vi "FaceEncoding.vi"(7 "numJitters":i32, 8 "error in (no error)":errorcluster, 9 "knownFaceLocation":refnum<k24>, 10 "image":refnum<k24>, 11 "FaceRecognition in":refnum<class "FaceRecognition.lvclass">) -> (0 "error out":errorcluster, 2 "FirstFaceEncoding":refnum<k24>, 3 "FaceRecognition out":refnum<class "FaceRecognition.lvclass">)   [LabVIEW 2020, in "FaceRecognitionDotNet.lvlib" / "FaceRecognition.lvclass"]
uses:
  FaceRecognition.lvclass
  dll/FaceRecognitionDotNet.dll
  FaceRecognition.lvclass/FaceRecognition.ctl
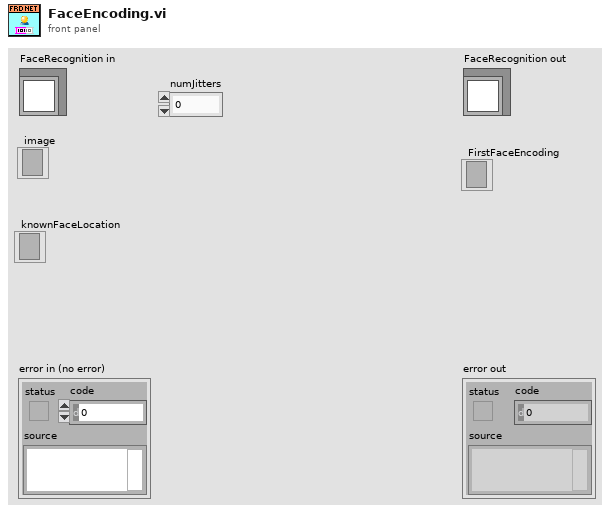
[diagram p1: front panel]
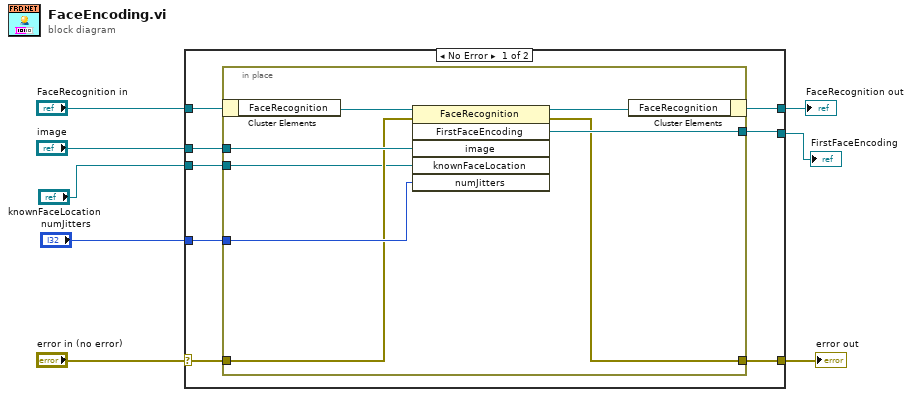
[diagram p0: block diagram]
diagram:
  n1 = case shown="No Error" "error in (no error)" {
    selector: "error in (no error)" -> [w14 w26]
    tunnel: [w13 w26] -> w7
    tunnel: [w15 w25] -> w5
    tunnel: "FaceRecognition in" -> [w16 w25]
    tunnel: [w12 _] -> w2
    tunnel: "image" -> [w11 _]
    tunnel: "numJitters" -> [w10 _]
    tunnel: "knownFaceLocation" -> [w9 _]
    frame No Error {
      n2 = in-place {
        in-place-border: w14 -> [w19]
        in-place-border: [w18] -> w13
        in-place-border: [w22] -> w12
        in-place-border: w11 -> [w21]
        in-place-border: w10 -> [w20]
        in-place-border: w9 -> [w17]
        n3 = in-place-cluster #1(w16) -> ("FaceRecognition"=w24:refnum<k24>)
        n4 = invoke class="FaceRecognition" method="FirstFaceEncoding"(reference=w24, error in=w19, "image"=w21, "knownFaceLocation"=w17, "numJitters"=w20) -> (reference out=w23:refnum<k24>, error out=w18:errorcluster, "FirstFaceEncoding"=w22:refnum<k24>)  [unwired: 1 in, 3 out]
        n5 = in-place-cluster #1("FaceRecognition"=w23) -> (w15:refnum<class "FaceRecognition.lvclass">)
      }
    }
    frame Error {
    }
  }
  "error out" <- w7
  "FaceRecognition out" <- w5
  "FirstFaceEncoding" <- w2
